vi "crc16-ccitt (xFFFF).vi"(8 "error in (no error)":errorcluster, 10 "Message":string) -> (0 "error out (dup)":errorcluster, 1 "Hex-Integer-String":string, 2 "CRC":u16 format="%.0x")   [LabVIEW 2020, in "Linearisierung v2.lvlib" / "Gasteiler.lvlib" / "HovaCal.lvlib"]
doc: "This VI takes in a string variable and calculates the 16-bit CRC value based on the CRC16-CCITT standard (polynomial 0x1021) with seed value of 0xFFFF ONLY!!!\n\nThis VI code is based on an extremely efficient implementation originally intended for microcontrollers and is adapted for LabVIEW. All thanks go to:\nOriginal Code: Ashley Roll\nOptimisations: Scott Dattalo"
uses:
  HovaCal.lvlib
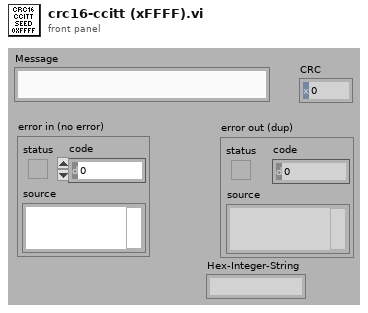
[diagram p1: front panel]
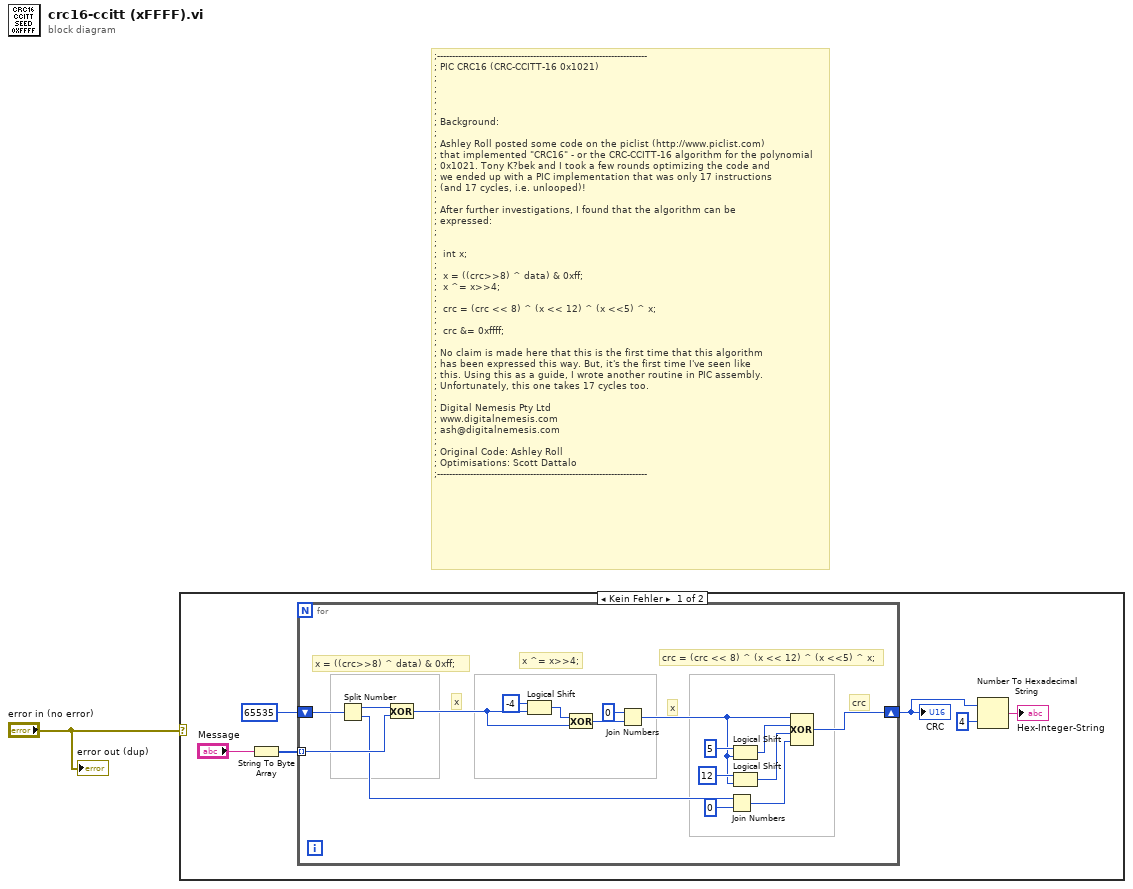
[diagram p0: block diagram]
diagram:
  # ";----------------------------------------------------------------------\n; PIC CRC16 (CRC-CCITT-16 0x1021)\n;\n;\n; \n;\n; Background:\n;\n; Ashley Roll posted some code on the piclist (http://www.piclist.com)\n; that implemented \"CRC16\" - or the CRC-CCITT-16 algorithm for the polynomial\n; 0x1021. Tony K?bek and I took a few rounds optimizing the code and\n; we ended up with a PIC implementation that was only 17 instructions\n; (and 17 cycles, i.e. unlooped)!\n;\n; After further investigations, I found that the algorithm can be \n; expressed:\n;\n;\n;  int x;\n;\n;  x = ((crc>>8) ^ data) & 0xff;\n;  x ^= x>>4;\n;\n;  crc = (crc << 8) ^ (x << 12) ^ (x <<5) ^ x;\n;\n;  crc &= 0xffff;\n;\n; No claim is made here that this is the first time that this algorithm\n; has been expressed this way. But, it's the first time I've seen like\n; this. Using this as a guide, I wrote another routine in PIC assembly.\n; Unfortunately, this one takes 17 cycles too.\n;\n; Digital Nemesis Pty Ltd\n; www.digitalnemesis.com\n; ash@digitalnemesis.com\n;\n; Original Code: Ashley Roll\n; Optimisations: Scott Dattalo\n;----------------------------------------------------------------------"
  n1 = case shown="Kein Fehler" "error in (no error)" {
    frame No Error {
      n2 = String To Byte Array(string="Message") -> (unsigned byte array=w6:u8[])
      n3 = for {
        tunnel: w6 -> [w18] mode=indexing
        shift-right: [w8] -> w4
        shift-left: u16 65535 -> [w17]
        # "crc"
        # "crc = (crc << 8) ^ (x << 12) ^ (x <<5) ^ x;"
        # "x"
        # "x ^= x>>4;"
        # "x"
        # "x = ((crc>>8) ^ data) & 0xff;"
        n4 = Split Number(x=w17) -> (hi(x)=w24:u8, lo(x)=w11:u8)
        n5 = Exclusive Or(1:w18, 2:w24) -> (0:w21:u8)
        n6 = Logical Shift(y=i8 -4, x=w21) -> (x << y=w22:u8)
        n7 = Exclusive Or(1:w21, 2:w22) -> (0:w20:u8)
        n8 = Join Numbers(hi=u8 0, lo=w20) -> ((hi.lo)=w13:u16)
        n9 = Join Numbers(hi=w11, lo=u8 0) -> ((hi.lo)=w9:u16)
        n10 = Logical Shift(y=i8 5, x=w13) -> (x << y=w15:u16)
        n11 = Logical Shift(y=i8 12, x=w13) -> (x << y=w12:u16)
        n12 = Compound Arithmetic op=XOR(w13, w15, w12, w9) -> (w8:u16)
      }
      "CRC" <- w4
      n13 = Number To Hexadecimal String(1:i16 4 ("Breite (-)"), 2:w4) -> (0:→"Hex-Integer-String":string)
    }
    frame Error {
    }
  }
  "error out (dup)" <- "error in (no error)"
